vi "Message - Timeout.vi"(8 "error in":errorcluster, 10 "Advice In":string="Tittle", 11 "Message In":string="Tittle") -> (0 "error out":errorcluster, 3 "Clamp Engaged?":bool)   [LabVIEW 2014]
panel:
  out "Warning":u16(ring)
  out "Advice Out":string="Tittle"
  out "Message Out":string="Tittle"
  in  "NO Button":bool
  in  "YES Button":bool
  # "ADVICE:"
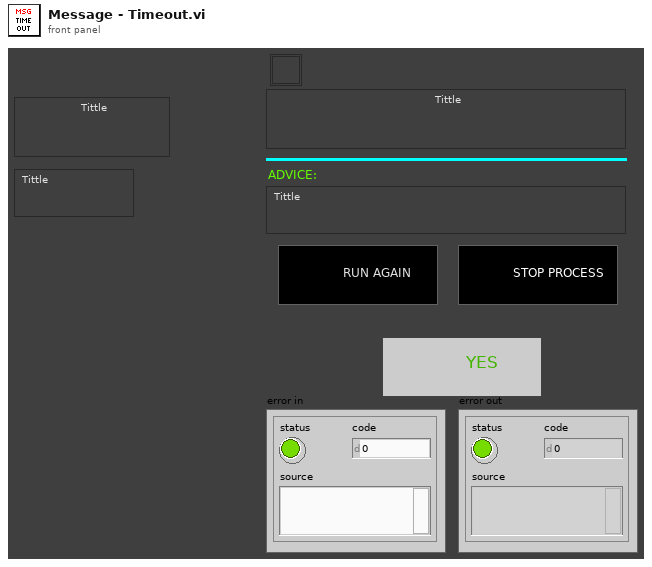
[diagram p1: front panel]
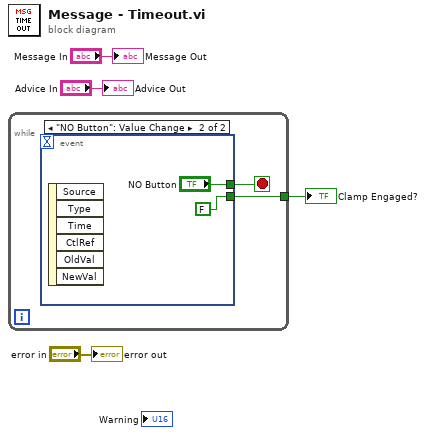
[diagram p0: block diagram]
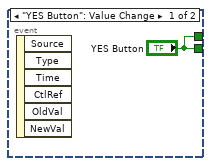
[diagram p2: hidden frame]
diagram:
  n1 = while {
    tunnel: [w6] -> w4
    stop <- w5 stop-if-true
    n2 = event shown="[1] \"NO Button\": Value Change" {
      selector: _ -> [_ _]
      dyn-events: _ -> [_ _]
      timeout: _ -> [_ _]
      tunnel: ["YES Button" "NO Button"] -> w5
      tunnel: ["YES Button" FALSE ("YES Button")] -> w6
      event "YES Button": Value Change {
        n3 = event-data() -> ()  [unwired: 1 in, 6 out]
      }
      event "NO Button": Value Change {
        n4 = event-data() -> ()  [unwired: 1 in, 6 out]
      }
    }
  }
  "Clamp Engaged?" <- w4
  "error out" <- "error in"
  "Message Out" <- "Message In"
  "Advice Out" <- "Advice In"
